vi "Size Test.vi"(5 "VI reference":refnum<vi>, 7 "Center Bounds":T1, 8 "error in":errorcluster, 11 "Editor Position in":refnum<class "Editor Position.lvclass">) -> (0 "error out":errorcluster, 3 "Editor Position out":refnum<class "Editor Position.lvclass">)   [LabVIEW 2021, in "Editor Position.lvclass"]
doc: "Tests the adjusting of the window size based on the Use Size flag."
uses:
  Editor Position.lvclass
  <vilib>/LabVIEW Icon API/lv_icon/lv_icon.lvlib
  <vilib>/Utility/miscctls.llb/LVRectTypeDef.ctl
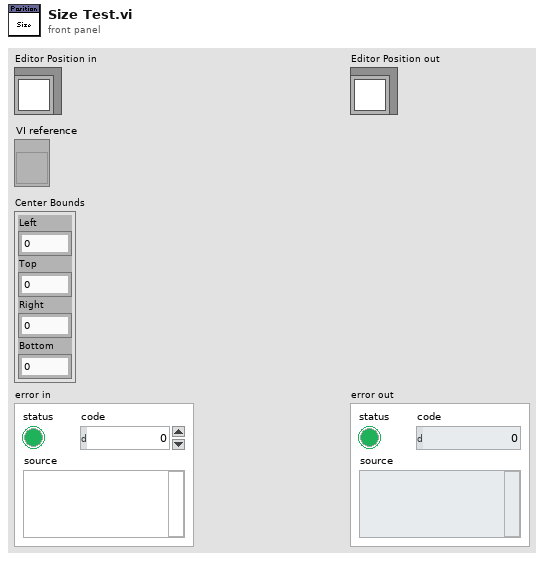
[diagram p1: front panel]
types:
  T1 = typedef "LVRectTypeDef.ctl" = cluster{"Left":i16, "Top":i16, "Right":i16, "Bottom":i16}
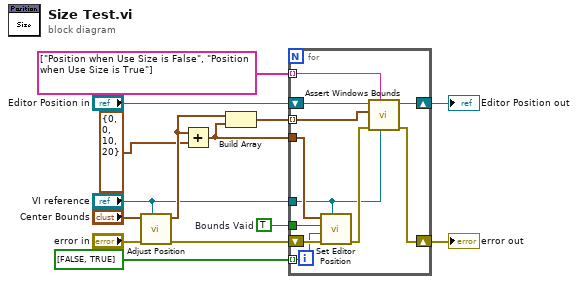
[diagram p0: block diagram]
diagram:
  w3 = TRUE  # Bounds Vaid
  n1 = call "Adjust Position.vi"("VI in"="VI reference", "error in"="error in", "Current Position"="Center Bounds") -> ("error out"=w12:errorcluster, "Adjusted Position"=w11:T1)  [unwired: 7 in]
  n2 = Add(x=w11, y=T1 {"Left"=0, "Top"=0, "Right"=10, "Bottom"=20}) -> (x+y=w2:T1)
  n3 = Build Array(w11, w2) -> (w4:T1[])
  n4 = for {
    tunnel: "VI reference" -> [w17]
    shift-right: [w19] -> w7
    shift-left: "Editor Position in" -> [w20]
    shift-right: [w23] -> w14
    shift-left: w12 -> [w25]
    tunnel: bool[] [FALSE, TRUE] -> [w21] mode=indexing
    tunnel: w4 -> [w18] mode=indexing
    tunnel: w3 -> [w16]
    tunnel: w2 -> [w22]
    tunnel: string[] ["Position when Use Size is False", "Position when Use Size is True"] -> [w15] mode=indexing
    n5 = call <resource>:"Set Editor Position.vi"("IE VI Ref"=w17, "error in"=w25, "Use Size"=w21, "Bounds Vaid"=w16, "Window Bounds"=w22) -> ("error out"=w24:errorcluster)  [unwired: 6 in]
    n6 = call "Assert Windows Bounds.vi"("VI reference"=w17, "Test Description"=w15, "error in"=w24, "Expected Position"=w18, "Editor Position in"=w20) -> ("error out"=w23:errorcluster, "Editor Position out"=w19:refnum<class "Editor Position.lvclass">)  [unwired: 5 in]
  }
  "error out" <- w14
  "Editor Position out" <- w7
